vi "OAT Easy Gabor Order Tracking (Analog Tach).vi"(0 "scaled signal [EU]":waveform(dbl)={"t0"=timestamp(0 s since 1904-01-01), "dt"=0.0, "Y"=[]}, 1 "bandwidth":T4={"bandwidth value"=0.5, "bandwidth unit"=enum."Order"} {"bandwidth value" min=0.0 format="%.2f"}, 2 "window info in (auto)":T1={"window type"=10, "window length"=0} {"window type" items=["None"=0, "Hanning"=1, "Hamming"=2, "Blackman-Harris"=3, "Exact Blackman"=4, "Blackman"=5, "Flat Top"=6, "4 Term B-Harris"=7, "7 Term B-Harris"=8, "Low Sidelobe"=9, "Gaussian"=62]; "window length" min=0}, 5 "orders (1.0)":dbl[](array[numeric])=[1.0] format="%.2f", 7 "analog tach signal":waveform(dbl)={"t0"=timestamp(0 s since 1904-01-01), "dt"=0.0, "Y"=[]}, 9 "pulse/revolution (1)":i32=1, 11 "error in (no error)":errorcluster, 12 "X axis selection":u16(ring)=2 items=["Time", "Revolution", "RPM"], 13 "phase setting":T2) -> (3 "samples/rev":dbl format="%.2f", 4 "magnitudes (RMS)":cluster{"X":dbl[], "Y":dbl[]}[](array[cluster]) {"Y" format="%.2f"; "X" format="%.2f"}, 6 "phase lags":cluster{"X":dbl[], "Y":dbl[]}[](array[cluster]) {"Y" format="%.2f"; "X" format="%.2f"}, 8 "order waveforms [EU]":waveform(dbl)[](array[waveform]), 10 "unit labels":T3, 15 "error out":errorcluster)   [LabVIEW 2017]
doc: "Extracts orders you designate from <B>scaled signal [EU]</B> and computes magnitudes and phase lags for the designated orders. You can use this polymorphic VI to perform order tracking for an analog tachometer signal or a digital tachometer signal. The data type you wire to the <B>analog tach signal</B> input determines the polymorphic instance to use."
uses:
  <vilib>/addons/Sound and Vibration/Order Analysis/Ref Gabor Order Tracking/Mask Bandwidth.ctl
  <vilib>/addons/Sound and Vibration/Order Analysis/Ref Gabor Order Tracking/window information.ctl
  <vilib>/addons/Sound and Vibration/Order Analysis/Tach Process/SubVIs/speed profile.ctl
  <vilib>/addons/Sound and Vibration/Order Analysis/Gabor Order Tracking/OAT Extract Order Waveforms (Single Order).vi
  <vilib>/addons/Sound and Vibration/Order Analysis/Tach Process/SoundVib_TachProcess.lvlib
  <vilib>/addons/Sound and Vibration/Order Analysis/Gabor Order Tracking/SoundVib_Gabor.lvlib
panel:
  # "OAT Easy Gabor Order Tracking (Analog Tach)"
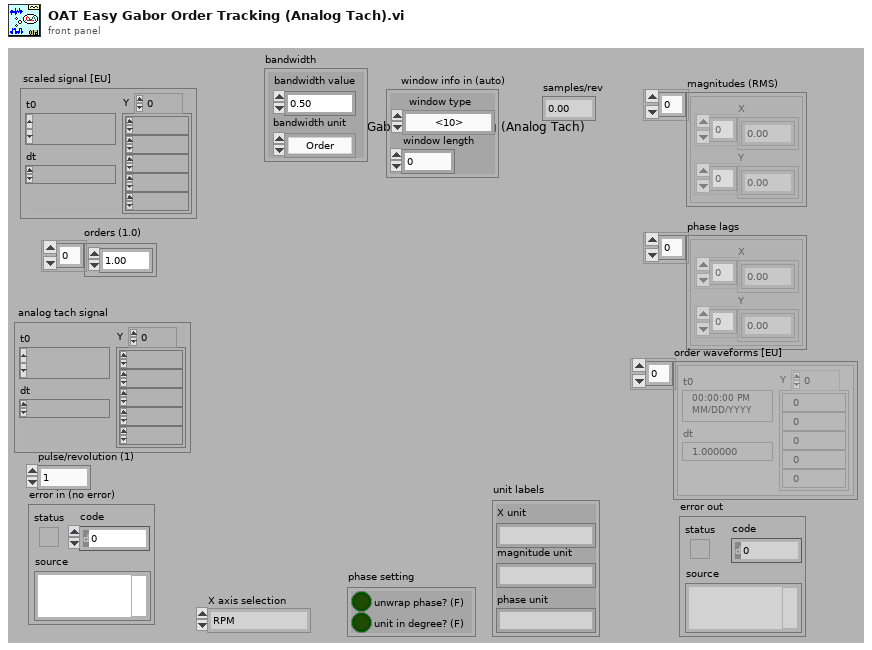
[diagram p1: front panel]
types:
  T1 = typedef "SoundVib_Gabor.lvlib/window information.ctl" = cluster{"window type":u32, "window length":i32}
  T2 = cluster{"unwrap phase? (F)":bool, "unit in degree? (F)":bool}
  T3 = cluster{"X unit":string, "magnitude unit":string, "phase unit":string}
  T4 = typedef "SoundVib_Gabor.lvlib/Mask Bandwidth.ctl" = cluster{"bandwidth value":dbl, "bandwidth unit":enum16{"Order", "Hz"}}
  T5 = typedef "SoundVib_TachProcess.lvlib/speed profile.ctl" = cluster{"time [s]":dbl[], "speed [RPM]":dbl[]}
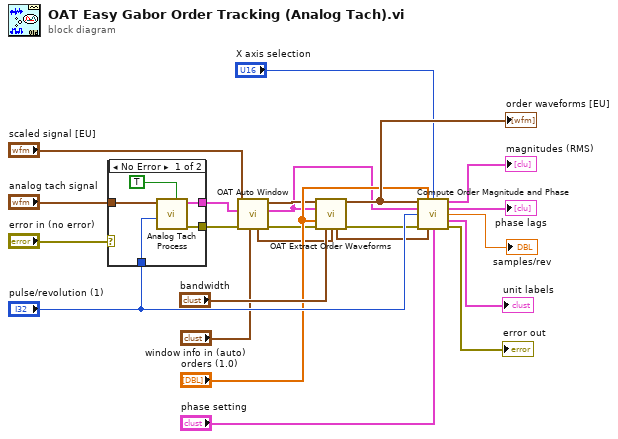
[diagram p0: block diagram]
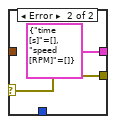
[diagram p2: hidden frame]
diagram:
  n1 = case shown="No Error" "error in (no error)" {
    selector: "error in (no error)" -> [_ w30]
    tunnel: "analog tach signal" -> [w28 _]
    tunnel: "pulse/revolution (1)" -> [w27 _]
    tunnel: [w26 T5 {"time [s]"=[], "speed [RPM]"=[]} ("speed profile")] -> w12
    tunnel: [w25 w30] -> w6
    frame No Error {
      n2 = call <vilib>:"Analog Tach Process.vi"("reset? (True)"=TRUE ("reset? (False)"), "pulse/revolution (1)"=w27, "analog tach signal"=w28) -> ("error out"=w25:errorcluster, "speed profile"=w26:T5)  [unwired: 6 in, 1 out]
    }
    frame Error {
    }
  }
  n3 = call <vilib>:"OAT Auto Window.vi"("window info in"="window info in (auto)", "error in (no error)"=w6, "speed profile"=w12, "scaled signal [EU]"="scaled signal [EU]") -> ("error out"=w7:errorcluster, "speed profile out"=w3:T5, "scaled signal [EU] out"=w11:waveform(dbl), "window info out"=w8:T1)  [unwired: 4 in]
  n4 = call-poly <vilib>:"OAT Extract Order Waveforms.vi"("scaled signal [EU]"=w11, "speed profile"=w3, "orders to extract"="orders (1.0)", "error in (no error)"=w7, "bandwidth"="bandwidth", "window info"=w8) -> ("order waveforms [EU]"=w21:waveform(dbl)[], "actual window info"=w10:T1, "error out"=w5:errorcluster)  [unwired: 6 in, 1 out]
  "order waveforms [EU]" <- w21
  n5 = call <vilib>:"Compute Order Magnitude and Phase.vi"("order waveforms [EU]"=w21, "orders (1.0)"="orders (1.0)", "X axis selection"="X axis selection", "speed profile"=w3, "pulse/revolution (1)"="pulse/revolution (1)", "error in (no error)"=w5, "window info"=w10, "phase setting"="phase setting") -> ("magnitudes (RMS)"=→"magnitudes (RMS)":cluster{"X":dbl[], "Y":dbl[]}[], "phase lags"=→"phase lags":cluster{"X":dbl[], "Y":dbl[]}[], "samples/rev"=→"samples/rev":dbl, "unit labels"=→"unit labels":T3, "error out"=→"error out":errorcluster)  [unwired: 3 in]
